vi "RSZVB Get TDIF Receiver Frequency.vi"(8 "error in (no error)":errorcluster {"code" format="%.0x"}, 9 "Channel (1)":i32=1, 11 "VISA session":refnum<visa-resource-name>) -> (0 "error out":errorcluster {"code" format="%.0x"}, 2 "Receiver Frequency":dbl format="%^.3e", 3 "dup VISA session":refnum<visa-resource-name>)   [LabVIEW 2011]
doc: "This VI returns the receiver frequency for true differential source adjustment.\n\nRemote-control command(s):\nSOURce<Ch>:TDIF:CRFRequency?"
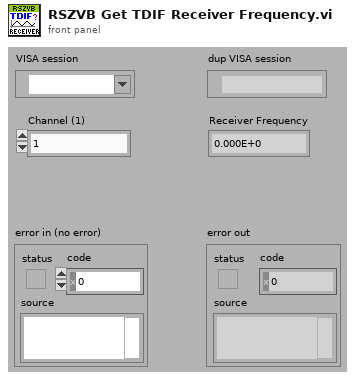
[diagram p1: front panel]
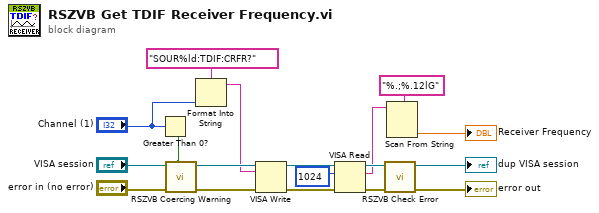
[diagram p0: block diagram]
diagram:
  n1 = Greater Than 0?(x="Channel (1)") -> (x > 0?=w7:bool)
  n2 = call "RSZVB Coercing Warning.vi"("In Range?"=w7, "error in (no error)"="error in (no error)", "VISA session"="VISA session") -> ("error out"=w10:errorcluster, "dup VISA session"=w11:refnum<visa-resource-name>)  [unwired: 7 in]
  n3 = Format Into String(format string="SOUR%ld:TDIF:CRFR?", "Channel (1)") -> (resulting string=w8:string)  [unwired: 2 in, 1 out]
  n4 = VISA Write(VISA resource name=w11, write buffer=w8, error in (no error)=w10) -> (VISA resource name out=w12:refnum<visa-resource-name>, error out=w13:errorcluster)  [unwired: 1 out]
  n5 = VISA Read(VISA resource name=w12, byte count=u32 1024 ("byte count (0)"), error in (no error)=w13) -> (VISA resource name out=w17:refnum<visa-resource-name>, read buffer=w14:string, error out=w16:errorcluster)  [unwired: 1 out]
  n6 = call "RSZVB Check Error.vi"("error in (no error)"=w16, "VISA session"=w17) -> ("error out"=→"error out":errorcluster, "dup VISA session"=→"dup VISA session":refnum<visa-resource-name>)  [unwired: 8 in]
  n7 = Scan From String(format string="%.;%.12lG", input string=w14) -> (output 1=→"Receiver Frequency":dbl)  [unwired: 3 in, 3 out]
